vi "Find Tests.vi"(8 "error in (no error)":errorcluster, 10 "File Paths":path[](array[path]), 11 "LUnit Test Suite":refnum<class "LUnit Test Suite.lvclass">) -> (0 "error out":errorcluster, 3 "LUnit Test Suite":refnum<class "LUnit Test Suite.lvclass">)   [LabVIEW 2020, in "Test Finder.lvclass"]
uses:
  Test Finder.lvclass
  API/LUnit Test Suite/LUnit Test Suite.lvclass
  C:/git/astemes-lunit/source/Core/Runnable/Runnable.lvclass
  Test Finder.lvclass/Test Finder.ctl
  API/Test Suite Factory/Test Suite Factory.lvclass
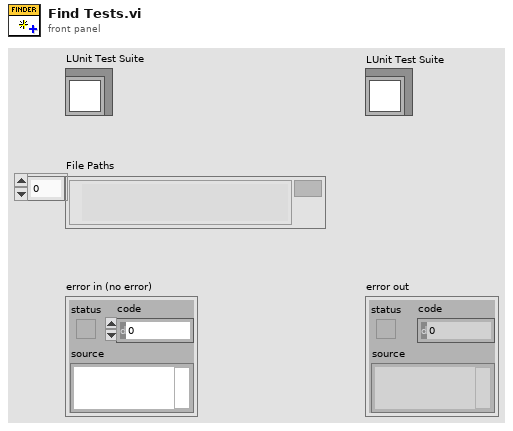
[diagram p1: front panel]
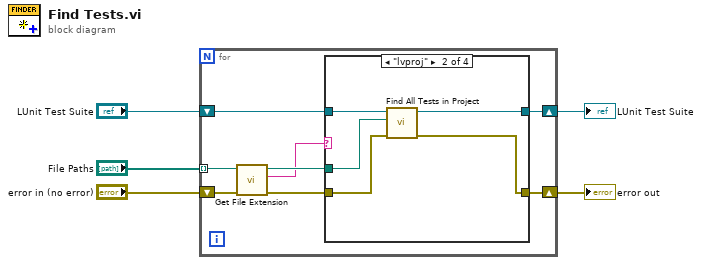
[diagram p0: block diagram]
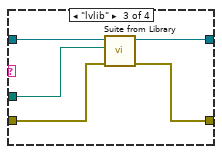
[diagram p3: hidden frame]
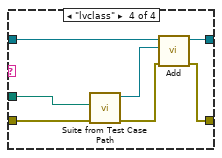
[diagram p4: hidden frame]
diagram:
  n1 = for {
    tunnel: "File Paths" -> [w8] mode=indexing
    shift-right: [w10] -> w4
    shift-left: "error in (no error)" -> [w13]
    shift-right: [w11] -> w3
    shift-left: "LUnit Test Suite" -> [w12]
    n2 = call <vilib>:"Get File Extension.vi"("error in (no error)"=w13, "file"=w8) -> ("error out"=w9:errorcluster, "lowercase file extension"=w6:string, "dup file"=w7:path)  [unwired: 5 in, 2 out]
    n3 = case shown="\"lvproj\"" w6 {
      tunnel: w12 -> [w15 w16 w21 w28]
      tunnel: [w15 w17 w22 w30] -> w11
      tunnel: [w14 w20 w25 w26] -> w10
      tunnel: w9 -> [w14 w19 w24 w32]
      tunnel: w7 -> [_ w18 w23 w31]
      frame Default {
      }
      frame "lvproj" {
        n4 = call "Find All Tests in Project.vi"("error in (no error)"=w19, "Projext Path"=w18, "LUnit Test Suite In"=w16) -> ("error out"=w20:errorcluster, "LUnit Test Suite out"=w17:refnum<class "LUnit Test Suite.lvclass">)  [unwired: 7 in]
      }
      frame "lvlib" {
        n5 = call "Suite from Library.vi"("error in (no error)"=w24, "Library Path"=w23, "LUnit Test Suite In"=w21) -> ("error out"=w25:errorcluster, "LUnit Test Suite Out"=w22:refnum<class "LUnit Test Suite.lvclass">)  [unwired: 7 in]
      }
      frame "lvclass" {
        n6 = call "Suite from Test Case Path.vi"("error in (no error)"=w32, "Test Case"=w31) -> ("error out"=w27:errorcluster, "LUnit Test Suite Out"=w29:refnum<class "LUnit Test Suite.lvclass">)  [unwired: 8 in]
        n7 = call "Add.vi"("error in (no error)"=w27, "Runnable"=w29, "LUnit Test Suite In"=w28) -> ("error out"=w26:errorcluster, "LUnit Test Suite Out"=w30:refnum<class "LUnit Test Suite.lvclass">)  [unwired: 7 in]
      }
    }
  }
  "error out" <- w4
  "LUnit Test Suite" <- w3
